vi "SP_GetXY.vi"(8 "error in (no error)":errorcluster, 11 "SemiProbe in":refnum<class "SemiProbe.lvclass">) -> (0 "error out":errorcluster, 1 "Y out":dbl, 2 "X out":dbl, 3 "SemiProbe out":refnum<class "SemiProbe.lvclass">)   [LabVIEW 2019, in "SemiProbe.lvclass"]
uses:
  SemiProbe.lvclass
  <vilib>/regexp/Match Regular Expression.xnode
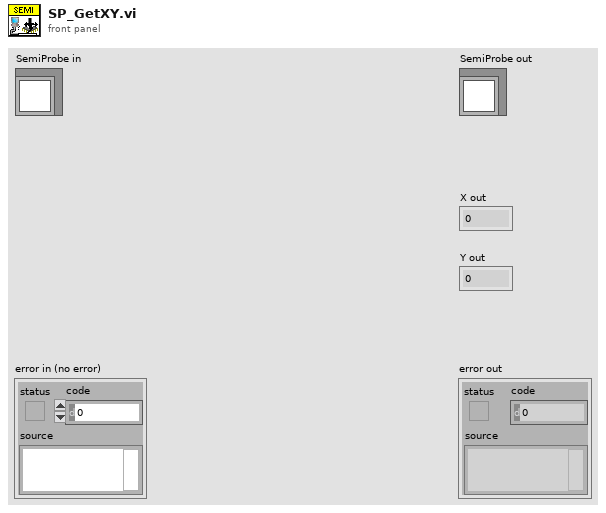
[diagram p1: front panel]
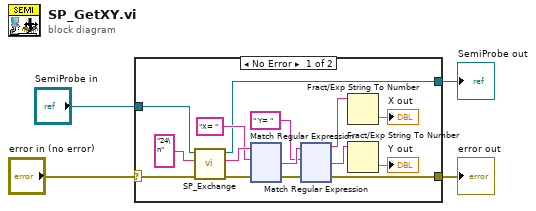
[diagram p0: block diagram]
diagram:
  n1 = case shown="No Error" "error in (no error)" {
    selector: "error in (no error)" -> [w10 w249]
    tunnel: [w9 w249] -> w3
    tunnel: [w7 w248] -> w1
    tunnel: "SemiProbe in" -> [w8 w248]
    frame No Error {
      n2 = call-dynamic "SP_Exchange.vi"("error in (no error)"=w10, "command"="24\n", "SemiProbe in"=w8) -> ("error out"=w13:errorcluster, "answer"=w17:string, "SemiProbe out"=w7:refnum<class "SemiProbe.lvclass">)  [unwired: 4 in, 2 out]
      n3 = xnode "Match Regular Expression"("input string"=w17, "regular expression"="X= ", "error in"=w13) -> ("after match"=w15:string, "error out"=w12:errorcluster)  [unwired: 3 in, 3 out]
      n4 = xnode "Match Regular Expression"("input string"=w15, "regular expression"=" Y= ", "error in"=w12) -> ("before match"=w18:string, "after match"=w19:string, "error out"=w9:errorcluster)  [unwired: 3 in, 2 out]
      n5 = Fract/Exp String To Number(string=w18) -> (number=→"X out":dbl)  [unwired: 3 in, 1 out]
      n6 = Fract/Exp String To Number(string=w19) -> (number=→"Y out":dbl)  [unwired: 3 in, 1 out]
    }
    frame Error {
    }
  }
  "error out" <- w3
  "SemiProbe out" <- w1
